vi "ntr.flow-panel.init.vi"(8 "error in (no error) 2":errorcluster, 11 "Controls in":refnum<vi>[](array[refnum])) -> (0 "error in (no error)":errorcluster, 2 "Elements Names":string[](array[string]), 3 "Controls out":refnum<vi>[](array[refnum]))   [LabVIEW 2024]
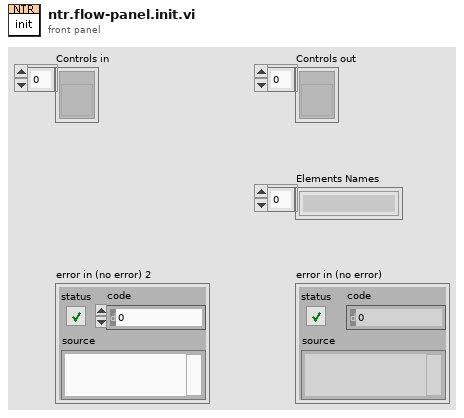
[diagram p1: front panel]
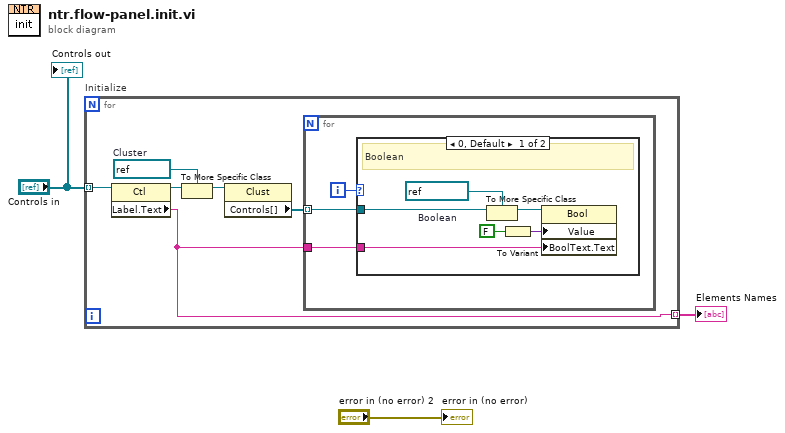
[diagram p0: block diagram]
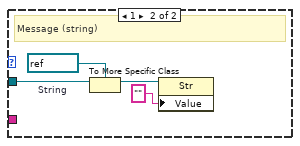
[diagram p2: hidden frame]
diagram:
  n1 = for "Initialize" {
    tunnel: "Controls in" -> [w9] mode=indexing
    tunnel: [w5] -> w3 mode=indexing
    w4 = refnum<vi> refnum  # Cluster
    n2 = property class="Ctl"(reference=w9) -> (reference out=w8:refnum<vi>, "Label.Text"=w5:string)  [unwired: 1 in, 1 out]
    n3 = To More Specific Class(target class=w4, reference=w8) -> (specific class reference=w7:refnum<vi>)  [unwired: 1 in, 1 out]
    n4 = property class="Clust"(reference=w7) -> ("Controls[]"=w6:refnum<vi>[])  [unwired: 1 in, 2 out]
    n5 = for {
      tunnel: w6 -> [w12] mode=indexing
      tunnel: w5 -> [w10]
      i -> [w11]
      n6 = case shown="0, Default" w11 {
        tunnel: w12 -> [w14 w20]
        tunnel: w10 -> [w13 _]
        frame 0, Default {
          w17 = refnum<vi> refnum  # Boolean
          # "Boolean"
          n7 = To More Specific Class(target class=w17, reference=w14) -> (specific class reference=w18:refnum<vi>)  [unwired: 1 in, 1 out]
          n8 = To Variant(anything=FALSE) -> (Variant=w15:variant)
          n9 = property class="Bool"(reference=w18, "Value"=w15, "BoolText.Text"=w13) -> ()  [unwired: 1 in, 2 out]
        }
        frame 1 {
          w21 = refnum<vi> refnum  # String
          # "Message (string)"
          n10 = To More Specific Class(target class=w21, reference=w20) -> (specific class reference=w22:refnum<vi>)  [unwired: 1 in, 1 out]
          n11 = property class="Str"(reference=w22, "Value"="" ("Boolean Text.Text")) -> ()  [unwired: 1 in, 2 out]
        }
      }
    }
  }
  "Elements Names" <- w3
  "error in (no error)" <- "error in (no error) 2"
  "Controls out" <- "Controls in"
